vi "Compare Parameters.vi"(9 "refresh listbox":T5[](array[typedef]), 10 "new parameter":T1={"name"="", "direction"=enum."Rx", "default value"=0.0, "unit"="", "Parameter"={"start index"=0, "size"=1, "encoding"=enum."BNR", "signed"=FALSE, "scale multiplier"=1.0, "scale offset"=0.0}}, 11 "old parameter":T1={"name"="", "direction"=enum."Rx", "default value"=0.0, "unit"="", "Parameter"={"start index"=0, "size"=1, "encoding"=enum."BNR", "signed"=FALSE, "scale multiplier"=1.0, "scale offset"=0.0}}) -> (1 "refresh listbox out":T5[](array[typedef]))   [LabVIEW 2020, in "Ballard ARINC 429 System Explorer.lvlib" / "Implementation.lvlib"]
uses:
  Implementation.lvlib
  Types/Refresh Listbox.ctl
  Types/Refresh Symbols.ctl
  Shared/VS Channel Definition for Parameter.ctl
  Shared/Direction.ctl
  Shared/Parameter Definition.ctl
  Encoding and Decoding/Encoding.ctl
  Encoding and Decoding/Encoding and Decoding.lvlib
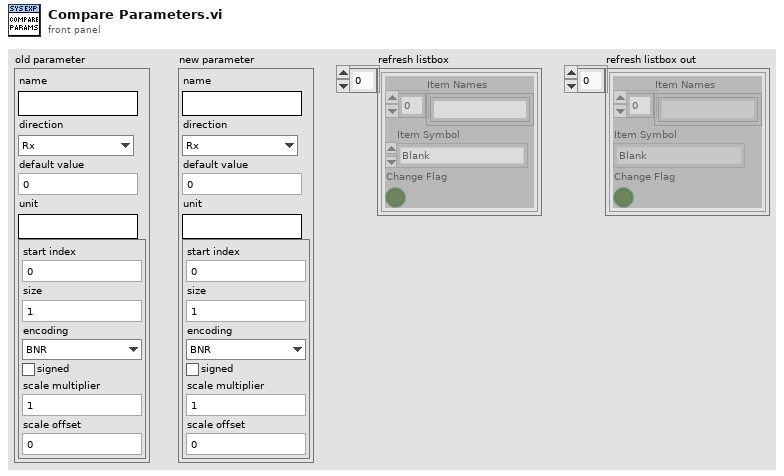
[diagram p1: front panel]
types:
  T1 = typedef "VS Channel Definition for Parameter.ctl" = cluster{"name":string, "direction":T2, "default value":dbl, "unit":string, "Parameter":T3}
  T2 = typedef "Direction.ctl" = enum16{"Rx", "Tx"}
  T3 = typedef "Parameter Definition.ctl" = cluster{"start index":i32, "size":i32, "encoding":T4, "signed":bool, "scale multiplier":dbl, "scale offset":dbl}
  T4 = typedef "Encoding and Decoding.lvlib/Encoding.ctl" = enum16{"BNR", "BCD", "Discrete"}
  T5 = typedef "Ballard ARINC 429 System Explorer.lvlib/Implementation.lvlib/Refresh Listbox.ctl" = cluster{"Item Names":string[], "Item Symbol":T6, "Change Flag":bool}
  T6 = typedef "Ballard ARINC 429 System Explorer.lvlib/Implementation.lvlib/Refresh Symbols.ctl" = enum16{"Blank", "Port", "Incoming", "Outgoing", "Label", "Word", "Parameter", "ARINC-429", "Config Files", "Channel Spec", "Item"}
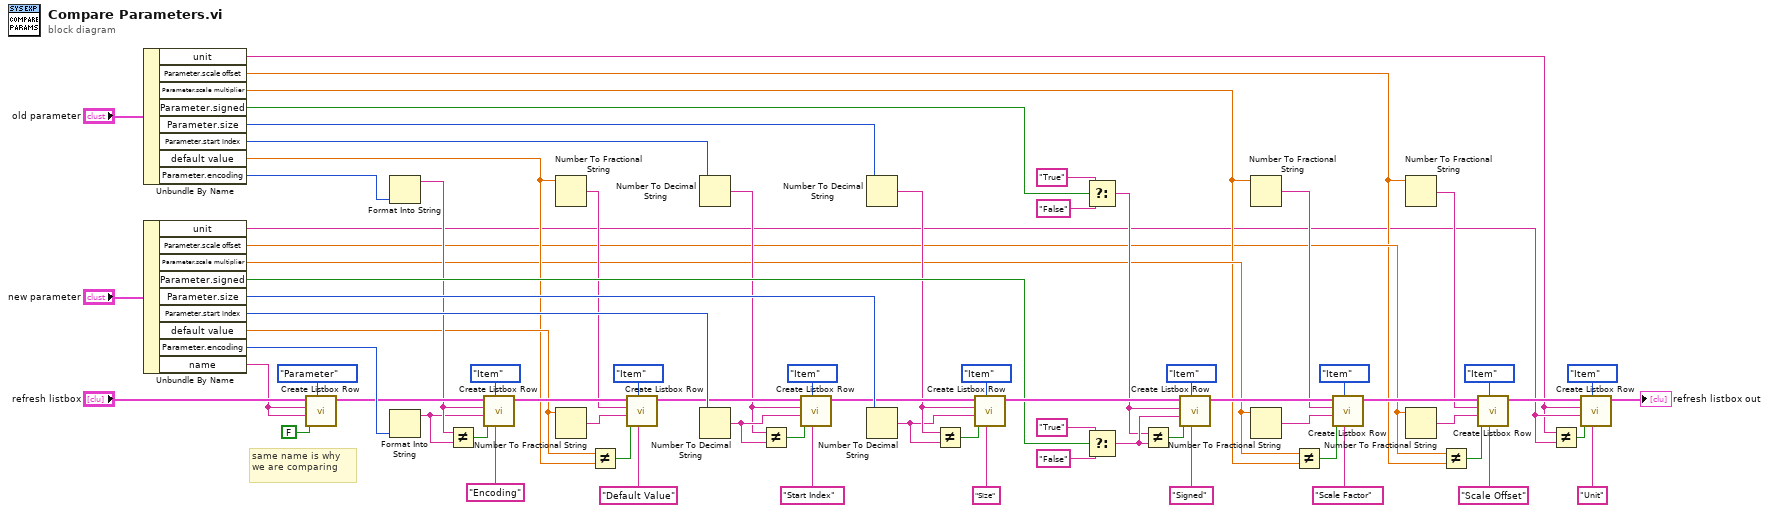
[diagram p0: block diagram]
diagram:
  # "same name is why we are comparing"
  n1 = Unbundle By Name("old parameter") -> ("unit"=w1:string, "Parameter.scale offset"=w5:dbl, "Parameter.scale multiplier"=w8:dbl, "Parameter.signed"=w15:bool, "Parameter.size"=w21:i32, "Parameter.start index"=w25:i32, "default value"=w26:dbl, "Parameter.encoding"=w33:T4)
  n2 = Unbundle By Name("new parameter") -> ("unit"=w2:string, "Parameter.scale offset"=w6:dbl, "Parameter.scale multiplier"=w9:dbl, "Parameter.signed"=w49:bool, "Parameter.size"=w56:i32, "Parameter.start index"=w60:i32, "default value"=w27:dbl, "Parameter.encoding"=w69:T4, "name"=w35:string)
  n3 = call "Create Listbox Row.vi"("refresh symbol (Blank)"=Refresh_Symbols."Parameter" ("Refresh Symbol (Blank)"), "change? (T)"=FALSE, "new item"=w35, "old item"=w35, "refresh listbox"="refresh listbox") -> ("refresh listbox out"=w67:T5[])  [unwired: 6 in]
  n4 = Format Into String(w33) -> (resulting string=w31:string)  [unwired: 3 in, 1 out]
  n5 = Format Into String(w69) -> (resulting string=w30:string)  [unwired: 3 in, 1 out]
  n6 = Not Equal?(x=w31, y=w30) -> (x != y?=w32:bool)
  n7 = call "Create Listbox Row.vi"("override name"="Encoding" ("name"), "refresh symbol (Blank)"=Refresh_Symbols."Item" ("Refresh Symbol (Blank)"), "change? (T)"=w32, "new item"=w30, "old item"=w31, "refresh listbox"=w67) -> ("refresh listbox out"=w63:T5[])  [unwired: 5 in]
  n8 = Number To Fractional String(number=w26) -> (F-format string=w29:string)  [unwired: 3 in]
  n9 = Number To Fractional String(number=w27) -> (F-format string=w64:string)  [unwired: 3 in]
  n10 = Not Equal?(x=w27, y=w26) -> (x != y?=w28:bool)
  n11 = call "Create Listbox Row.vi"("override name"="Default Value" ("name"), "refresh symbol (Blank)"=Refresh_Symbols."Item" ("Refresh Symbol (Blank)"), "change? (T)"=w28, "new item"=w64, "old item"=w29, "refresh listbox"=w63) -> ("refresh listbox out"=w59:T5[])  [unwired: 5 in]
  n12 = Number To Decimal String(number=w25) -> (decimal integer string=w22:string)  [unwired: 1 in]
  n13 = Number To Decimal String(number=w60) -> (decimal integer string=w23:string)  [unwired: 1 in]
  n14 = Not Equal?(x=w22, y=w23) -> (x != y?=w24:bool)
  n15 = call "Create Listbox Row.vi"("override name"="Start Index" ("name"), "refresh symbol (Blank)"=Refresh_Symbols."Item" ("Refresh Symbol (Blank)"), "change? (T)"=w24, "new item"=w23, "old item"=w22, "refresh listbox"=w59) -> ("refresh listbox out"=w55:T5[])  [unwired: 5 in]
  n16 = Number To Decimal String(number=w21) -> (decimal integer string=w19:string)  [unwired: 1 in]
  n17 = Number To Decimal String(number=w56) -> (decimal integer string=w18:string)  [unwired: 1 in]
  n18 = Not Equal?(x=w19, y=w18) -> (x != y?=w20:bool)
  n19 = call "Create Listbox Row.vi"("override name"="Size" ("name"), "refresh symbol (Blank)"=Refresh_Symbols."Item" ("Refresh Symbol (Blank)"), "change? (T)"=w20, "new item"=w18, "old item"=w19, "refresh listbox"=w55) -> ("refresh listbox out"=w50:T5[])  [unwired: 5 in]
  n20 = Select(t="True", s=w15, f="False") -> (s? t:f=w12:string)
  n21 = Select(t="True", s=w49, f="False") -> (s? t:f=w13:string)
  n22 = Not Equal?(x=w12, y=w13) -> (x != y?=w14:bool)
  n23 = call "Create Listbox Row.vi"("override name"="Signed" ("name"), "refresh symbol (Blank)"=Refresh_Symbols."Item" ("Refresh Symbol (Blank)"), "change? (T)"=w14, "new item"=w13, "old item"=w12, "refresh listbox"=w50) -> ("refresh listbox out"=w45:T5[])  [unwired: 5 in]
  n24 = Number To Fractional String(number=w8) -> (F-format string=w11:string)  [unwired: 3 in]
  n25 = Number To Fractional String(number=w9) -> (F-format string=w48:string)  [unwired: 3 in]
  n26 = Not Equal?(x=w9, y=w8) -> (x != y?=w10:bool)
  n27 = call "Create Listbox Row.vi"("override name"="Scale Factor" ("name"), "refresh symbol (Blank)"=Refresh_Symbols."Item" ("Refresh Symbol (Blank)"), "change? (T)"=w10, "new item"=w48, "old item"=w11, "refresh listbox"=w45) -> ("refresh listbox out"=w41:T5[])  [unwired: 5 in]
  n28 = Number To Fractional String(number=w5) -> (F-format string=w4:string)  [unwired: 3 in]
  n29 = Number To Fractional String(number=w6) -> (F-format string=w42:string)  [unwired: 3 in]
  n30 = Not Equal?(x=w6, y=w5) -> (x != y?=w7:bool)
  n31 = call "Create Listbox Row.vi"("override name"="Scale Offset" ("name"), "refresh symbol (Blank)"=Refresh_Symbols."Item" ("Refresh Symbol (Blank)"), "change? (T)"=w7, "new item"=w42, "old item"=w4, "refresh listbox"=w41) -> ("refresh listbox out"=w39:T5[])  [unwired: 5 in]
  n32 = Not Equal?(x=w1, y=w2) -> (x != y?=w3:bool)
  n33 = call "Create Listbox Row.vi"("override name"="Unit" ("name"), "refresh symbol (Blank)"=Refresh_Symbols."Item" ("Refresh Symbol (Blank)"), "change? (T)"=w3, "new item"=w2, "old item"=w1, "refresh listbox"=w39) -> ("refresh listbox out"=→"refresh listbox out":T5[])  [unwired: 5 in]
